vi "Begin Map.vi"   [LabVIEW 2019, in "LabPack.lvlib" / "Reader.lvclass"]
doc: "Begins reading a map. This does not decode the contents of the map, it just tells the internal decoder to start decoding a series of key-value pairs (map)."
uses:
  Reader.lvclass
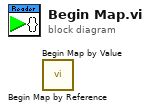
[diagram p0: block diagram]
diagram:
  n1 = call "Begin Map by Reference.vi"() -> ()  [unwired: 9 in, 3 out]
  n2 = call "Begin Map by Value.vi"() -> ()  [unwired: 9 in, 3 out]
